vi "Right Front Rocket Backup.vi"() -> (4 "path":cluster{"X":dbl, "Y":dbl}[](array[cluster])=[{"X"=200.0, "Y"=26.0}, {"X"=199.19449822516654, "Y"=26.59180599281069}, {"X"=198.38901421431035, "Y"=27.183607700427814}, {"X"=197.58359880252704, "Y"=27.77541039357613}, {"X"=196.7783030316455, "Y"=28.367223405888826}, {"X"=195.97317181624243, "Y"=28.959054905188317}, {"X"=195.16824839211316, "Y"=29.55090929258512}, {"X"=194.36358525427113, "Y"=30.14278854085464}, {"X"=193.55925438744458, "Y"=30.734695627317976}, {"X"=192.75535265213858, "Y"=31.326637407276202}, {"X"=191.95200314972453, "Y"=31.918625489181537}, {"X"=191.1493564574656, "Y"=32.51067541990231}, {"X"=190.347595544053, "Y"=33.10280551061733}, {"X"=189.54694603733955, "Y"=33.695036569935915}, {"X"=188.7476912597159, "Y"=34.287393059005645}, {"X"=187.95019046451995, "Y"=34.879905391475845}, {"X"=187.15489926715733, "Y"=35.47261272150291}, {"X"=186.36239274908786, "Y"=36.06556568220824}, {"X"=185.57339323173858, "Y"=36.65882895899089}, {"X"=184.7888056507876, "Y"=37.25248402267786}, {"X"=184.00976368797183, "Y"=37.846632603120185}, {"X"=183.23768963350713, "Y"=38.441401503395106}, {"X"=182.4743708236443, "Y"=39.0369492162953}, {"X"=181.72205581851014, "Y"=39.633474647561634}, {"X"=180.9835745048689, "Y"=40.23122813719044}, {"X"=180.26248696555496, "Y"=40.83052525012114}, {"X"=179.56327535756233, "Y"=41.43176362434687}, {"X"=178.8915570957225, "Y"=42.03544236549305}, {"X"=178.25444236569228, "Y"=42.642194916728336}, {"X"=177.66077732448244, "Y"=43.25280422349881}, {"X"=177.12178782374087, "Y"=43.86827153351722}, {"X"=176.65152623277436, "Y"=44.48984401147633}, {"X"=176.26764096973082, "Y"=45.119086526190344}, {"X"=175.9923618758584, "Y"=45.75797385325141}, {"X"=175.85364260596828, "Y"=46.40898939943156}, {"X"=175.85806178492393, "Y"=47.09620183415102}, {"X"=175.9763197277428, "Y"=47.81220233606906}, {"X"=176.18512174089372, "Y"=48.551099989625754}, {"X"=176.46595027168368, "Y"=49.30821140947831}, {"X"=176.80407541970908, "Y"=50.07981138150617}, {"X"=177.1877725708644, "Y"=50.86293531939989}, {"X"=177.60771096216018, "Y"=51.655224174321916}, {"X"=178.05647139481985, "Y"=52.45480190675955}, {"X"=178.5281583811361, "Y"=53.26017729757312}, {"X"=179.01808571367116, "Y"=54.07016474394593}, {"X"=179.52252443487126, "Y"=54.88382086586293}, {"X"=180.03850481402688, "Y"=55.700394517394216}, {"X"=180.5636623872591, "Y"=56.519287702220666}, {"X"=181.0961170702137, "Y"=57.340024811103994}, {"X"=181.63437594032493, "Y"=58.1622279684049}, {"X"=182.17725364178852, "Y"=58.985596974720714}, {"X"=182.72380747039, "Y"=59.80989299944634}, {"X"=183.27328571868813, "Y"=60.63492554961037}, {"X"=183.82508781680747, "Y"=61.46054230092281}, {"X"=184.37873408266407, "Y"=62.28662127896226}, {"X"=184.9338424397882, "Y"=63.11306480323294}, {"X"=185.4901097043667, "Y"=63.939794649843456}, {"X"=186.0472958342066, "Y"=64.7667480443341}, {"X"=186.60521052799456, "Y"=65.59387419558823}, {"X"=187.16370157062775, "Y"=66.4211318892354}, {"X"=187.72264740009558, "Y"=67.24848483925615}, {"X"=188.2819465204417, "Y"=68.07590787119182}, {"X"=188.84151823621482, "Y"=68.90336446282492}, {"X"=189.40129754560652, "Y"=69.73084494839156}, {"X"=189.9612193237363, "Y"=70.5583129862759}, {"X"=190.52124418313488, "Y"=71.3857479622073}, {"X"=191.08132952488273, "Y"=72.21313013239858}, {"X"=191.64142932900504, "Y"=73.04042737187049}, {"X"=192.20150617707017, "Y"=73.86760380551104}, {"X"=192.7615246355387, "Y"=74.69462268330884}, {"X"=193.32144012666078, "Y"=75.52143880455836}, {"X"=193.88119856603782, "Y"=76.34799263492167}, {"X"=194.44074058312682, "Y"=77.17420973385036}, {"X"=195.0, "Y"=78.0}], 6 "Reverse Path?":bool=TRUE)   [LabVIEW 2018]
uses:
  AutonBuilder/Typedef/Data Point.ctl
panel:
  in  "Data Points":T1[](array[typedef])=[{"X"=200.0, "Y"=26.0, "Theta"=0.0, "Speed %"=0.0, "Disabled?"=FALSE}, {"X"=173.13402061855672, "Y"=45.721254355400696, "Theta"=0.0, "Speed %"=0.0, "Disabled?"=FALSE}, {"X"=195.0, "Y"=78.0, "Theta"=0.0, "Speed %"=0.0, "Disabled?"=FALSE}]
  out "Graph":cluster{dbl[], dbl[]}[](graph)=[{[180.5, 214.0, 214.0, 180.5, 180.5], [40.25, 40.25, 11.75, 11.75, 40.25]}, {[200.0, 173.13402061855672, 195.0], [26.0, 45.721254355400696, 78.0]}, {[200.0, 199.19449822516654, 198.38901421431035, 197.58359880252704, 196.7783030316455, 195.97317181624243, 195.16824839211316, 194.36358525427113, 193.55925438744458, 192.75535265213858, 191.95200314972453, 191.1493564574656, 190.347595544053, 189.54694603733955, 188.7476912597159, 187.95019046451995, 187.15489926715733, 186.36239274908786, 185.57339323173858, 184.7888056507876, 184.00976368797183, 183.23768963350713, 182.4743708236443, 181.72205581851014, 180.9835745048689, 180.26248696555496, 179.56327535756233, 178.8915570957225, 178.25444236569228, 177.66077732448244, 177.12178782374087, 176.65152623277436, 176.26764096973082, 175.9923618758584, 175.85364260596828, 175.85806178492393, 175.9763197277428, 176.18512174089372, 176.46595027168368, 176.80407541970908, 177.1877725708644, 177.60771096216018, 178.05647139481985, 178.5281583811361, 179.01808571367116, 179.52252443487126, 180.03850481402688, 180.5636623872591, 181.0961170702137, 181.63437594032493, 182.17725364178852, 182.72380747039, 183.27328571868813, 183.82508781680747, 184.37873408266407, 184.9338424397882, 185.4901097043667, 186.0472958342066, 186.60521052799456, 187.16370157062775, 187.72264740009558, 188.2819465204417, 188.84151823621482, 189.40129754560652, 189.9612193237363, 190.52124418313488, 191.08132952488273, 191.64142932900504, 192.20150617707017, 192.7615246355387, 193.32144012666078, 193.88119856603782, 194.44074058312682, 195.0], [26.0, 26.59180599281069, 27.183607700427814, 27.77541039357613, 28.367223405888826, 28.959054905188317, 29.55090929258512, 30.14278854085464, 30.734695627317976, 31.326637407276202, 31.918625489181537, 32.51067541990231, 33.10280551061733, 33.695036569935915, 34.287393059005645, 34.879905391475845, 35.47261272150291, 36.06556568220824, 36.65882895899089, 37.25248402267786, 37.846632603120185, 38.441401503395106, 39.0369492162953, 39.633474647561634, 40.23122813719044, 40.83052525012114, 41.43176362434687, 42.03544236549305, 42.642194916728336, 43.25280422349881, 43.86827153351722, 44.48984401147633, 45.119086526190344, 45.75797385325141, 46.40898939943156, 47.09620183415102, 47.81220233606906, 48.551099989625754, 49.30821140947831, 50.07981138150617, 50.86293531939989, 51.655224174321916, 52.45480190675955, 53.26017729757312, 54.07016474394593, 54.88382086586293, 55.700394517394216, 56.519287702220666, 57.340024811103994, 58.1622279684049, 58.985596974720714, 59.80989299944634, 60.63492554961037, 61.46054230092281, 62.28662127896226, 63.11306480323294, 63.939794649843456, 64.7667480443341, 65.59387419558823, 66.4211318892354, 67.24848483925615, 68.07590787119182, 68.90336446282492, 69.73084494839156, 70.5583129862759, 71.3857479622073, 72.21313013239858, 73.04042737187049, 73.86760380551104, 74.69462268330884, 75.52143880455836, 76.34799263492167, 77.17420973385036, 78.0]}, {[201.86128028735055, 207.6316686140757, 206.82626576798532, 206.0213261550025, 205.21693992330364, 204.41309963435222, 203.60980239162532, 202.80714146552015, 202.0053312207689, 201.20467450812524, 200.40551834308292, 199.60823885612433, 198.81326834952338, 198.0211511415912, 197.2326054807507, 196.44857617241425, 195.67027755266173, 194.89923907730778, 194.13737076226153, 193.38706347171944, 192.65133370992334, 191.9340188115678, 191.24002928557402, 190.57567130992996, 189.9490628648075, 189.37067347705857, 188.85409222395856, 188.41673801903946, 188.08182998273307, 187.8778118761488, 187.8420720085181, 188.01560156610492, 188.43251061041937, 189.0792497003343, 189.79075672360892, 190.1077671579137, 190.0358426997249, 189.89811276070094, 189.82647248254307, 189.8558977798234, 189.9843511625043, 190.19845843464958, 190.48307158277208, 190.82446523392952, 191.21115003932024, 191.63382493820723, 192.08505857257137, 192.5589355281452, 193.0507523422548, 193.55677762969114, 194.07406230087227, 194.60028263791457, 195.13360691855195, 195.67258429956215, 196.2160574790317, 196.7630985718771, 197.31296390871472, 197.86506128573322, 198.4189227018597, 198.97418541099023, 199.53054622073444, 200.08782004060566, 200.6457374100227, 201.20424947311562, 201.76317237371904, 202.32236669621554, 202.88181497023461, 203.4414383219709, 204.00112555073045, 204.56082414004516, 205.1205121789647, 205.68013428681635, 206.23959926734528, 206.79881579500872], [11.872079569451126, 38.07556216527075, 38.66730424030597, 39.25875734145188, 39.84990198759379, 40.44078467143418, 41.031443516797864, 41.62185028419753, 42.21190287148596, 42.80145593193908, 43.3903551266712, 43.97844802689367, 44.565566257955616, 45.15149098878101, 45.73591832043917, 46.31843415875435, 46.89849704853687, 47.475419089170046, 48.04833240983098, 48.616130552062, 49.177376954472784, 49.73017286376956, 50.27197176762113, 50.79931508749678, 51.307442222689396, 51.78969668192489, 52.23654136176875, 52.63418891299001, 52.96134956352154, 53.18631845412515, 53.256455969158395, 53.087535086316606, 52.540571999129995, 51.396756263451735, 49.37872845730553, 47.00456787218066, 45.49006672411445, 44.67600292107553, 44.352513047679764, 44.360332989203265, 44.593160495055436, 44.98172598491615, 45.48041248769312, 46.058556800633156, 46.695093059508984, 47.37523244207156, 48.088361770322145, 48.82669891329299, 49.58443356913729, 50.35717588930911, 51.14159010774578, 51.935133473265765, 52.73585718453964, 53.54225163366921, 54.35313057122156, 55.16755038556071, 55.98475734869083, 56.80415300674087, 57.625266746788256, 58.447740424084785, 59.27126568459107, 60.095691682021794, 60.92070139235109, 61.74630828075023, 62.572299950598904, 63.398507673392835, 64.22494865886918, 65.0515421075846, 65.87814308298782, 66.70468956700842, 67.53116980379622, 68.35752231979399, 69.18362566572101, 70.00935260223221]}, {[198.13871971264945, 190.7573278362574, 189.95176266063538, 189.14587145005157, 188.33966613998734, 187.53324399813263, 186.726694392601, 185.9200290430221, 185.11317755412026, 184.30603079615193, 183.49848795636615, 182.69047405880684, 181.88192273858263, 181.0727409330879, 180.26277703868112, 179.45180475662565, 178.63952098165294, 177.82554642086794, 177.00941570121563, 176.19054782985575, 175.36819366602032, 174.54136045544647, 173.7087123617146, 172.86844032709033, 172.0180861449303, 171.15430045405134, 170.2724584911661, 169.36637617240555, 168.4270547486515, 167.44374277281608, 166.40150363896365, 165.2874508994438, 164.10277132904227, 162.9054740513825, 161.91652848832763, 161.60835641193415, 161.9167967557607, 162.4721307210865, 163.1054280608243, 163.75225305959475, 164.3911939792245, 165.0169634896708, 165.62987120686762, 166.2318515283427, 166.82502138802207, 167.4112239315353, 167.9919510554824, 168.56838924637296, 169.14148179817258, 169.71197425095872, 170.28044498270478, 170.84733230286542, 171.4129645188243, 171.9775913340528, 172.54141068629644, 173.10458630769932, 173.66725550001865, 174.22953038268, 174.7914983541294, 175.35321773026527, 175.91474857945673, 176.47607300027772, 177.03729906240696, 177.59834561809743, 178.15926627375353, 178.72012167005423, 179.28084407953085, 179.84142033603916, 180.4018868034099, 180.96222513103226, 181.52236807435685, 182.0822628452593, 182.64188189890837, 183.20118420499128], [40.127920430548876, 15.108049820350631, 15.699911160549659, 16.292063445700382, 16.884544824183862, 17.477325138942454, 18.07037506837238, 18.66372679751175, 19.25748838314999, 19.851818882613323, 20.44689585169187, 21.04290281291095, 21.640044763279043, 22.238582151090817, 22.83886779757212, 23.44137662419734, 24.046728394468957, 24.655712275246433, 25.2693255081508, 25.888837493293725, 26.515888251767585, 27.15263014302065, 27.801926664969464, 28.46763420762649, 29.155014051691488, 29.871353818317395, 30.62698588692499, 31.43669581799608, 32.323040269935134, 33.31928999287248, 34.48008709787605, 35.89215293663605, 37.69760105325069, 40.11919144305108, 43.439250341557596, 47.18783579612138, 50.13433794802368, 52.42619705817598, 54.26390977127686, 55.79928977380907, 57.13271014374434, 58.32872236372768, 59.429191325825975, 60.46179779451309, 61.44523642838288, 62.3924092896543, 63.31242726446629, 64.21187649114835, 65.0956160530707, 65.96728004750068, 66.82960384169566, 67.68465252562692, 68.5339939146811, 69.37883296817641, 70.22011198670296, 71.05857922090517, 71.89483195099609, 72.72934308192733, 73.5624816443882, 74.39452335438601, 75.22570399392123, 76.05612406036184, 76.88602753329876, 77.7153816160329, 78.54432602195288, 79.37298825102177, 80.20131160592797, 81.02931263615639, 81.85706452803426, 82.68455579960926, 83.5117078053205, 84.33846295004935, 85.16479380197971, 85.99064739776779]}, {[], []}, {[], []}, {[], []}, {[], []}, {[], []}]
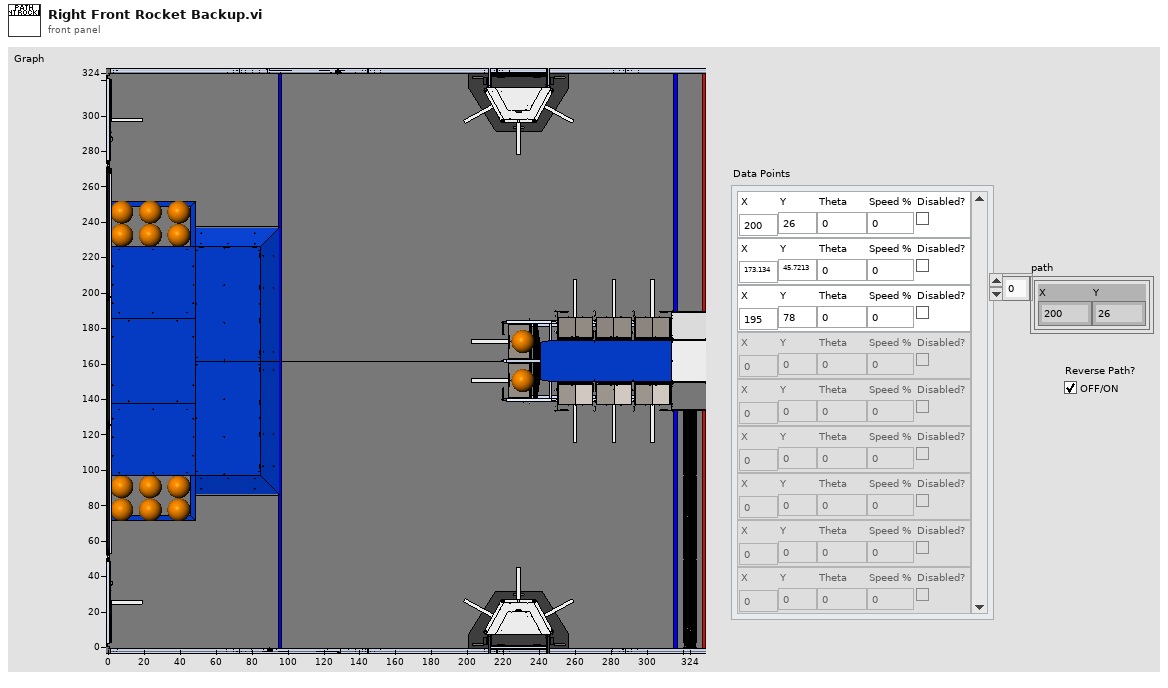
[diagram p1: front panel]
types:
  T1 = typedef "Data Point.ctl" = cluster{"X":dbl, "Y":dbl, "Theta":dbl, "Speed %":dbl, "Disabled?":bool}
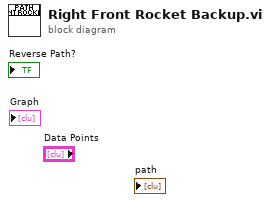
[diagram p0: block diagram]
diagram:
